vi "Laser Data Transfer.vi"(11 "VISA resource name":refnum<visa-resource-name>="COM3") -> (0 "error out":errorcluster, 3 "Laser Data Read":dbl)   [LabVIEW 2019]
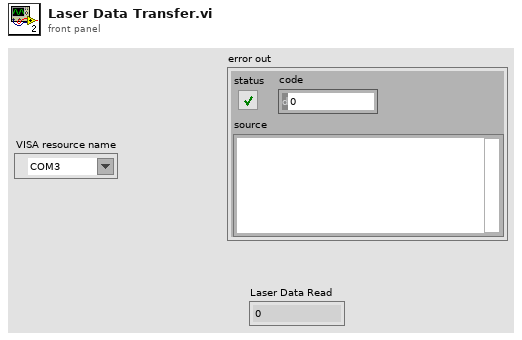
[diagram p1: front panel]
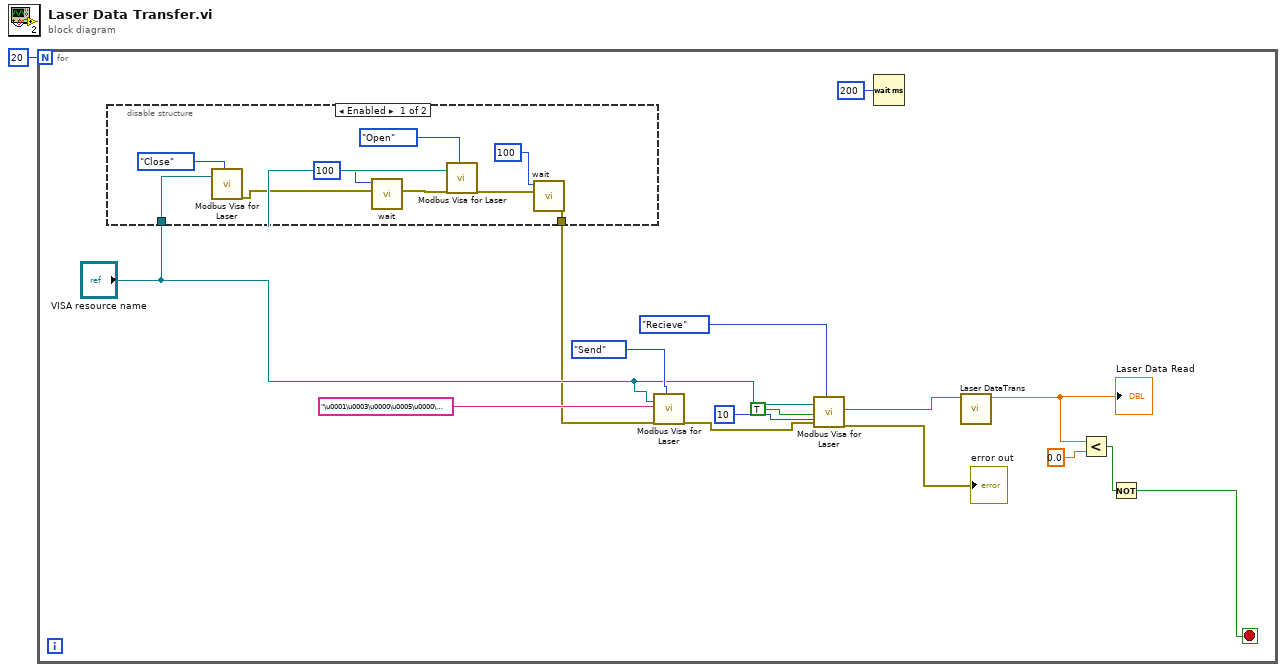
[diagram p0: block diagram]
diagram:
  n1 = for {
    N: 20 -> [_]
    stop <- w2 stop-if-true
    n2 = disable-structure shown="Enabled" {
      disable-tunnel: "VISA resource name" -> [w23 _]
      disable-tunnel: [w17 _] -> w7
      frame Enabled {
        n3 = call "Modbus Visa for Laser.vi"("VISA resource name"=w23, "VisaAction"=enum16{"Open", "Send", "Recieve", "Close"}."Close") -> ("error out"=w22:errorcluster)  [unwired: 16 in, 1 out]
        n4 = call "wait.vi"("error in"=w22, "wait(ms)"=u32 100) -> ("error out"=w20:errorcluster)  [unwired: 9 in]
        n5 = call "Modbus Visa for Laser.vi"("VISA resource name"=w23, "error in (no error)"=w20, "VisaAction"=enum16{"Open", "Send", "Recieve", "Close"}."Open") -> ("error out"=w18:errorcluster)  [unwired: 15 in, 1 out]
        n6 = call "wait.vi"("error in"=w18, "wait(ms)"=u32 100) -> ("error out"=w17:errorcluster)  [unwired: 9 in]
      }
      frame Disabled {
      }
    }
    n7 = call "Modbus Visa for Laser.vi"("VISA resource name"="VISA resource name", "Cmd"="\u0001\u0003\u0000\u0005\u0000\u0002Ô\n", "error in (no error)"=w7, "VisaAction"=enum16{"Open", "Send", "Recieve", "Close"}."Send") -> ("error out"=w14:errorcluster)  [unwired: 14 in, 1 out]
    n8 = call "Modbus Visa for Laser.vi"("VISA resource name"="VISA resource name", "TimeOut"=TRUE, "Time(0.1)"=u32 10, "error in (no error)"=w14, "VisaAction"=enum16{"Open", "Send", "Recieve", "Close"}."Recieve") -> ("read string"=w10:string, "error out"=→"error out":errorcluster)  [unwired: 13 in]
    n9 = Wait (ms)(milliseconds to wait=u32 200) -> ()  [unwired: 1 out]
    n10 = call "Laser DataTrans.vi"("Strin"=w10) -> ("Read"=w6:dbl)  [unwired: 10 in]
    "Laser Data Read" <- w6
    n11 = Less?(x=w6, y=0.0) -> (x < y?=w3:bool)
    n12 = Not(x=w3) -> (.not. x?=w2:bool)
  }
